vi "zlgcan_demo_PCIECANFD-200U.vi"() -> ()   [LabVIEW 2018]
doc: "用于设置CAN通道的初始化参数。\n\n适用的设备：PCIE-CANFD-100U、PCIE-CANFD-200U、PCIE-CANFD-400U。"
uses:
  data_type/ZCAN_Transmit_Data.ctl
  data_type/ZCAN_TransmitFD_Data.ctl
  data_type/ZCAN_InitCAN_setting_PCIEFD.ctl
panel:
  in  "PCIECANFD系列初始化参数":T1
  out "source":string
  in  "开启CAN":bool
  out "CANFD报文显示":string[][](table)
  in  "stop":bool
  in  "?":enum32{"DEMO说明", "设备、通道选择", "参数设置", "状态", "发送"}(tab)
  in  "CAN 通道":u32(ring) items=["0", "1"]
  in  "CAN卡型号":u32(ring)=39 items=["PCIE-CANFD-200U"=39]
  in  "索引":u32(ring) items=["0", "1", "2", "3", "4", "5", "6", "7", "8"]
  in  "仲裁域波特率":u32(ring)=500000 items=["1Mbps"=1000000, "800kbps"=800000, "500kbps"=500000, "250kbps"=250000, "125kbps"=125000, "100kbps"=100000, "50kbps"=50000]
  in  "数据域波特率":u32(ring)=1000000 items=["8Mbps"=8000000, "5Mbps"=5000000, "4Mbps"=4000000, "2Mbps"=2000000, "1Mbps"=1000000]
  in  "自定义波特率字符输入":string
  in  "自定义波特率开关":bool
  in  "验收码":u32
  in  "屏蔽码":u32=4294967295 format="%x"
  in  "滤波模式":u8(ring) items=["双滤波", "单滤波"]
  in  "工作模式":u8(ring) items=["正常", "只听"]
  out "error out":errorcluster caption="错误输出"
  out "can_index_handle(out)":u32
  out "Device_handle(out)":u32
  in  "帧类型":u32(ring) items=["标准帧", "扩展帧"]
  in  "发送方式":u32(ring) items=["正常发送", "单次发送", "自发自收", "单次自发自收"]
  in  "帧格式":u32(ring) items=["数据帧", "远程帧"]
  out "数据长度":u8=8 max=8
  in  "ID":u32=18 format="0x%08x"
  in  "协议":u32(ring) items=["CAN", "CANFD"]
  in  "数据输入":string="11 22 33 44 55 66 77 88"
  in  "CANFD加速？":u32(ring) items=["不加速", "加速"]
  in  "发送":bool
  in  "CANFD数据帧数组":T2(array[cluster])
  in  "CAN数据帧数组":T3(array[cluster])
  out "CAN报文显示":string[][](table)
  in  "ZCAN_TransmitFD_Data":T4
  in  "ZCAN_Transmit_Data":T5
  out "已接收帧数":u32
  # "适用的设备：PCIE-CANFD-200U。"
  # "停止程序前，\n请先关闭CAN卡"
  # "1. 确保电脑有VC++ 2005/2008/2010/2013运行库（对应32，64位）,微软常用运行库合集，点击下载（35M）。\n    http://manual.zlg.cn/Public/Uploads/2020-06-05/5ed995c271414.zip"
  # "2，如果打开设备失败，可能原因：\n（1）已经打开过一次，没有正常关闭的情况下，继续点击“打开设备”，是无法打开的。\n     需要USB重新拔插，LABVIEW重启（全部关闭），然后再“打开设备”。\n (2) 项目路径不能有中文繁体。"
  # "默认可以不设置"
  # "使用CAN时，\n只需要设置仲裁域波特率"
  # "使用ZCANPro软件波特率计算工具计算"
  # "CANFD数据长度只能是1~8，12，16，20，24，32，48，64"
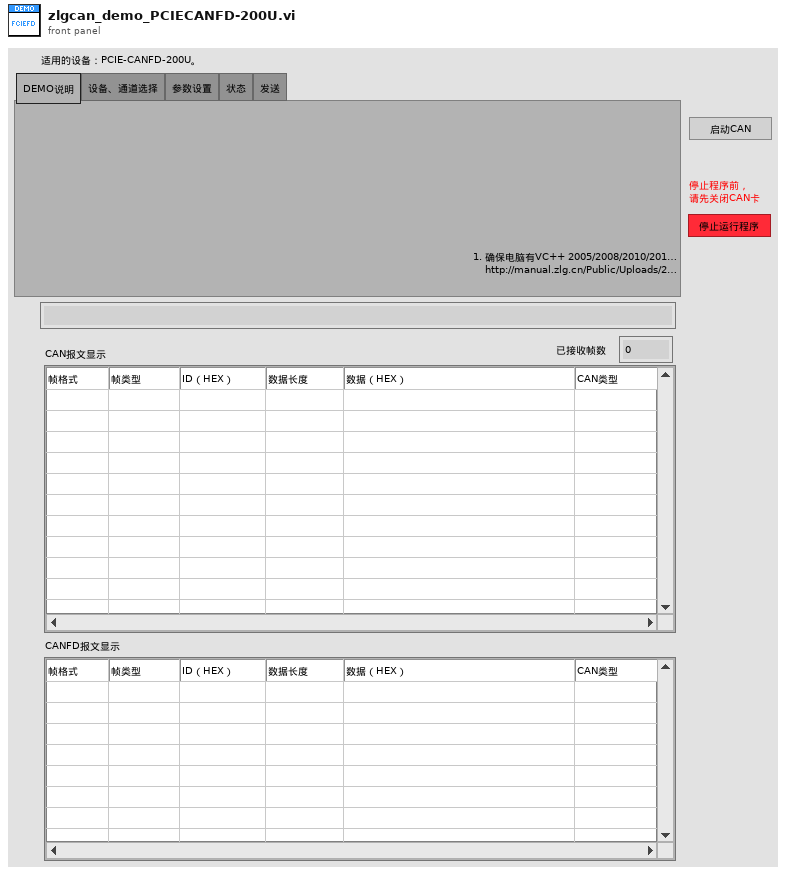
[diagram p1: front panel]
types:
  T1 = typedef "ZCAN_InitCAN_setting_PCIEFD.ctl" = cluster{"abitbaud":u32, "dbitbaud":u32, "baud_rate_custom？":bool, "RateCustom":string, "filter":u8, "acc_code":u32, "acc_mask":u32, "mode":u8}
  T2 = cluster{u32, u8, u8, u8, u8, cluster{"[0]":u8, "[1]":u8, "[2]":u8, "[3]":u8, "[4]":u8, "[5]":u8, "[6]":u8, "[7]":u8, "[8]":u8, "[9]":u8, "[10]":u8, "[11]":u8, "[12]":u8, "[13]":u8, "[14]":u8, "[15]":u8, "[16]":u8, "[17]":u8, "[18]":u8, "[19]":u8, "[20]":u8, "[21]":u8, "[22]":u8, "[23]":u8, "[24]":u8, "[25]":u8, "[26]":u8, "[27]":u8, "[28]":u8, "[29]":u8, "[30]":u8, "[31]":u8, "[32]":u8, "[33]":u8, "[34]":u8, "[35]":u8, "[36]":u8, "[37]":u8, "[38]":u8, "[39]":u8, "[40]":u8, "[41]":u8, "[42]":u8, "[43]":u8, "[44]":u8, "[45]":u8, "[46]":u8, "[47]":u8, "[48]":u8, "[49]":u8, "[50]":u8, "[51]":u8, "[52]":u8, "[53]":u8, "[54]":u8, "[55]":u8, "[56]":u8, "[57]":u8, "[58]":u8, "[59]":u8, "[60]":u8, "[61]":u8, "[62]":u8, "[63]":u8}, u64}[]
  T3 = cluster{u32, u8, u8, u8, u8, cluster{"[0]":u8, "[1]":u8, "[2]":u8, "[3]":u8, "[4]":u8, "[5]":u8, "[6]":u8, "[7]":u8}, u64}[]
  T4 = typedef "ZCAN_TransmitFD_Data.ctl" = cluster{"帧类型":u32, "帧格式":u32, "ID":u32, "数据长度":u8, "CANFD加速？":u8, "DATA":cluster{"CAN数据[0]":u8, "CAN数据[1]":u8, "CAN数据[2]":u8, "CAN数据[3]":u8, "CAN数据[4]":u8, "CAN数据[5]":u8, "CAN数据[6]":u8, "CAN数据[7]":u8, "CAN数据[8]":u8, "CAN数据[9]":u8, "CAN数据[10]":u8, "CAN数据[11] ":u8, "CAN数据[12] ":u8, "CAN数据[13] ":u8, "CAN数据[14] ":u8, "CAN数据[15] ":u8, "CAN数据[16]":u8, "CAN数据[17]":u8, "CAN数据[18]":u8, "CAN数据[19]":u8, "CAN数据[20]":u8, "CAN数据[21]":u8, "CAN数据[22]":u8, "CAN数据[23]":u8, "CAN数据[24] ":u8, "CAN数据[25]":u8, "CAN数据[26]":u8, "CAN数据[27]":u8, "CAN数据[28]":u8, "CAN数据[29]":u8, "CAN数据[30]":u8, "CAN数据[31]":u8, "CAN数据[32]":u8, "CAN数据[33]":u8, "CAN数据[34]":u8, "CAN数据[35]":u8, "CAN数据[36]":u8, "CAN数据[37]":u8, "CAN数据[38]":u8, "CAN数据[39]":u8, "CAN数据[40]":u8, "CAN数据[41]":u8, "CAN数据[42]":u8, "CAN数据[43]":u8, "CAN数据[44]":u8, "CAN数据[45]":u8, "CAN数据[46]":u8, "CAN数据[47]":u8, "CAN数据[48]":u8, "CAN数据[49]":u8, "CAN数据[50]":u8, "CAN数据[51]":u8, "CAN数据[52]":u8, "CAN数据[53]":u8, "CAN数据[54]":u8, "CAN数据[55]":u8, "CAN数据[56]":u8, "CAN数据[57]":u8, "CAN数据[58]":u8, "CAN数据[59]":u8, "CAN数据[60]":u8, "CAN数据[61]":u8, "CAN数据[62]":u8, "CAN数据[63]":u8}, "发送方式":u32}
  T5 = typedef "ZCAN_Transmit_Data.ctl" = cluster{"帧类型":u32, "帧格式":u32, "ID":u32, "数据长度":u8, "DATA":cluster{"CAN数据[0]":u8, "CAN数据[1]":u8, "CAN数据[2]":u8, "CAN数据[3]":u8, "CAN数据[4]":u8, "CAN数据[5]":u8, "CAN数据[6]":u8, "CAN数据[7]":u8}, "发送方式":u32}
  T6 = cluster{"[0]":u32, "[1]":u32, "[2]":u32, "[3]":u32, "[4]":u32, "[5]":u32, "[6]":u32, "[7]":u32, "[8]":u32, "[9]":u32, "[10]":u32, "[11]":u32, "[12]":u32, "[13]":u32, "[14]":u32, "[15]":u32, "[16]":u32, "[17]":u32, "[18]":u32, "[19]":u32, "[20]":u32, "[21]":u32, "[22]":u32, "[23]":u32, "[24]":u32, "[25]":u32, "[26]":u32, "[27]":u32, "[28]":u32, "[29]":u32, "[30]":u32, "[31]":u32, "[32]":u32, "[33]":u32, "[34]":u32, "[35]":u32, "[36]":u32, "[37]":u32, "[38]":u32, "[39]":u32, "[40]":u32, "[41]":u32, "[42]":u32, "[43]":u32, "[44]":u32, "[45]":u32, "[46]":u32, "[47]":u32, "[48]":u32, "[49]":u32, "[50]":u32, "[51]":u32, "[52]":u32, "[53]":u32, "[54]":u32, "[55]":u32, "[56]":u32, "[57]":u32, "[58]":u32, "[59]":u32, "[60]":u32, "[61]":u32, "[62]":u32, "[63]":u32}
  T7 = cluster{"[0]":u32, "[1]":u32, "[2]":u32, "[3]":u32, "[4]":u32, "[5]":u32, "[6]":u32, "[7]":u32}
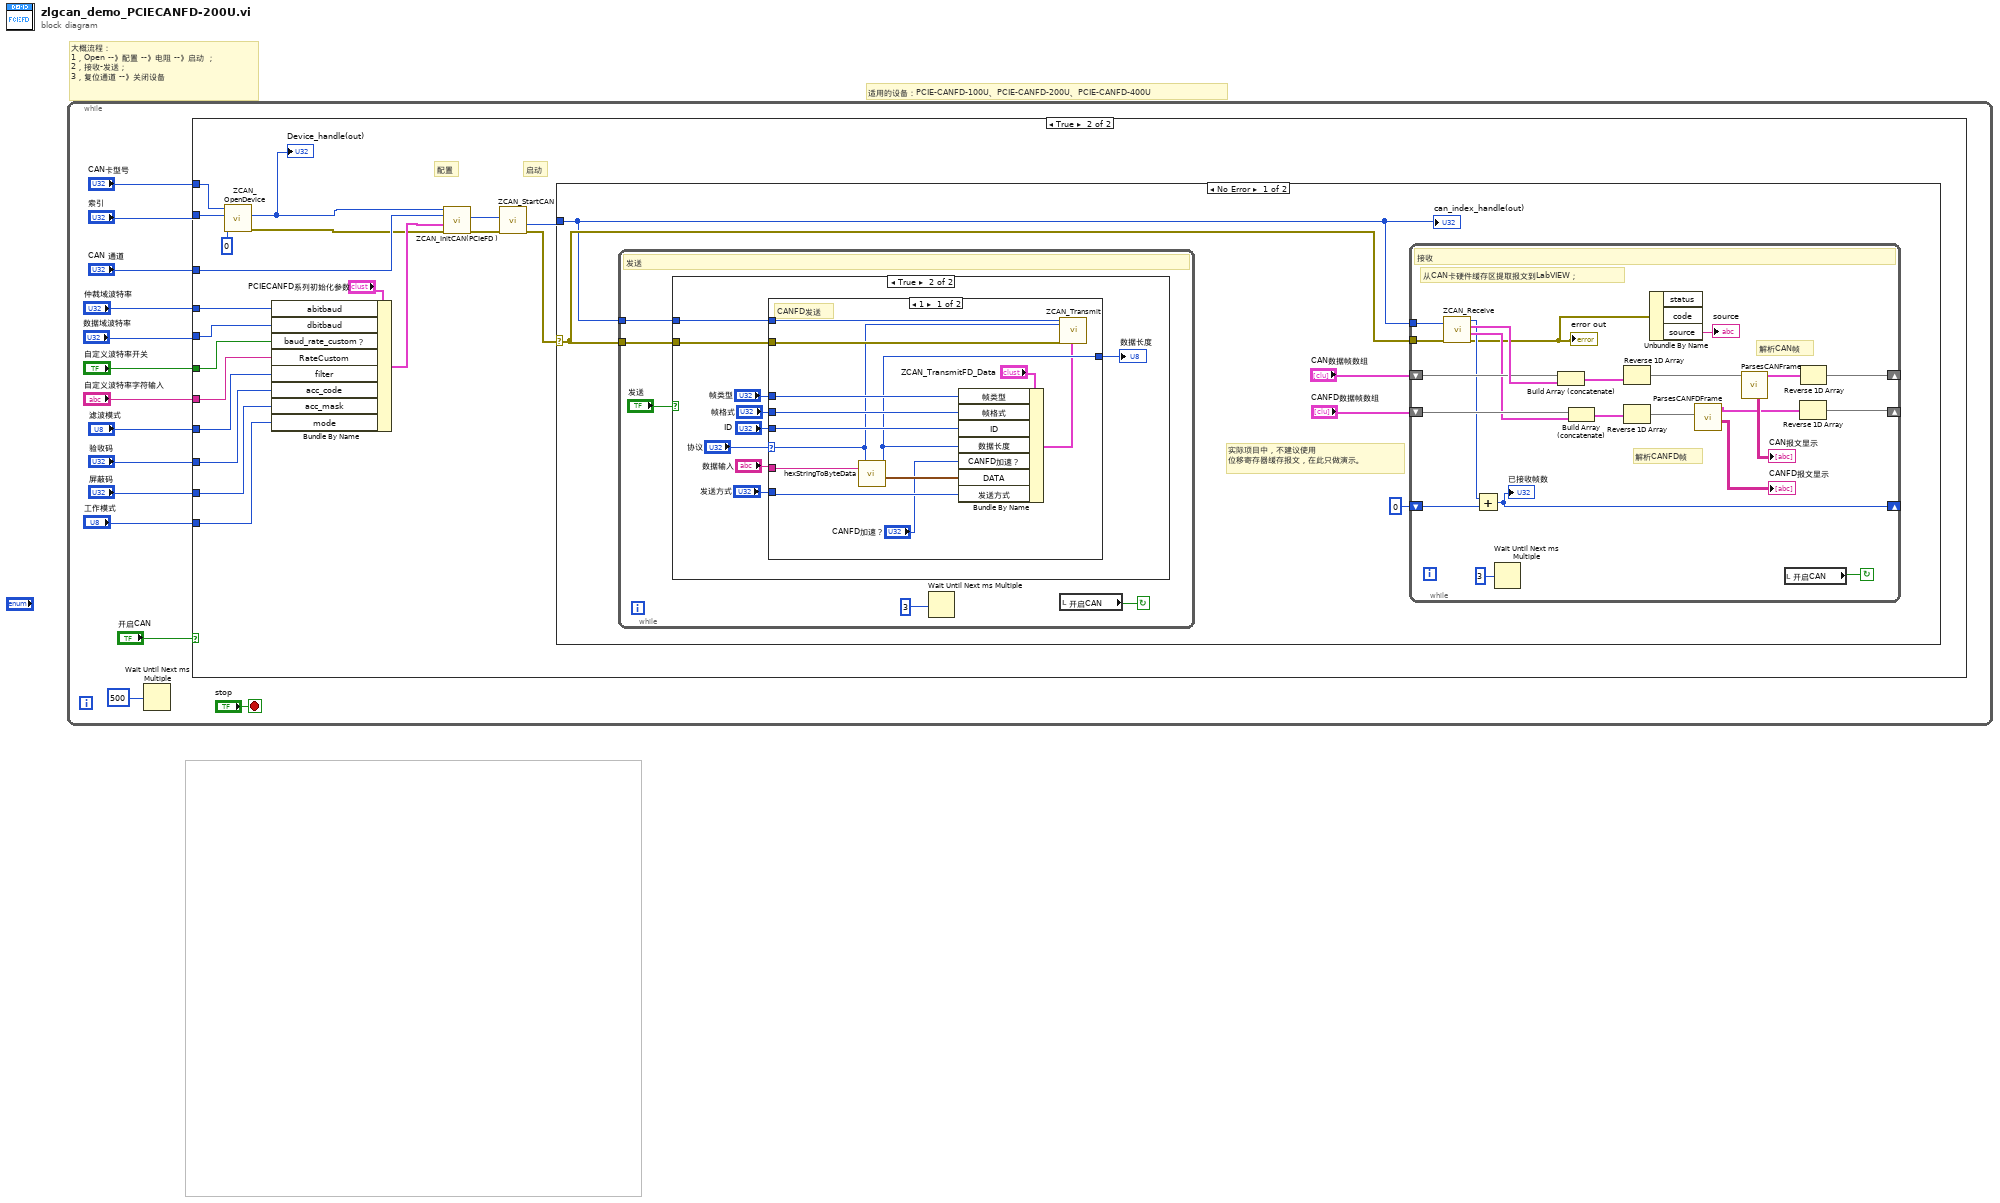
[diagram p0: block diagram]
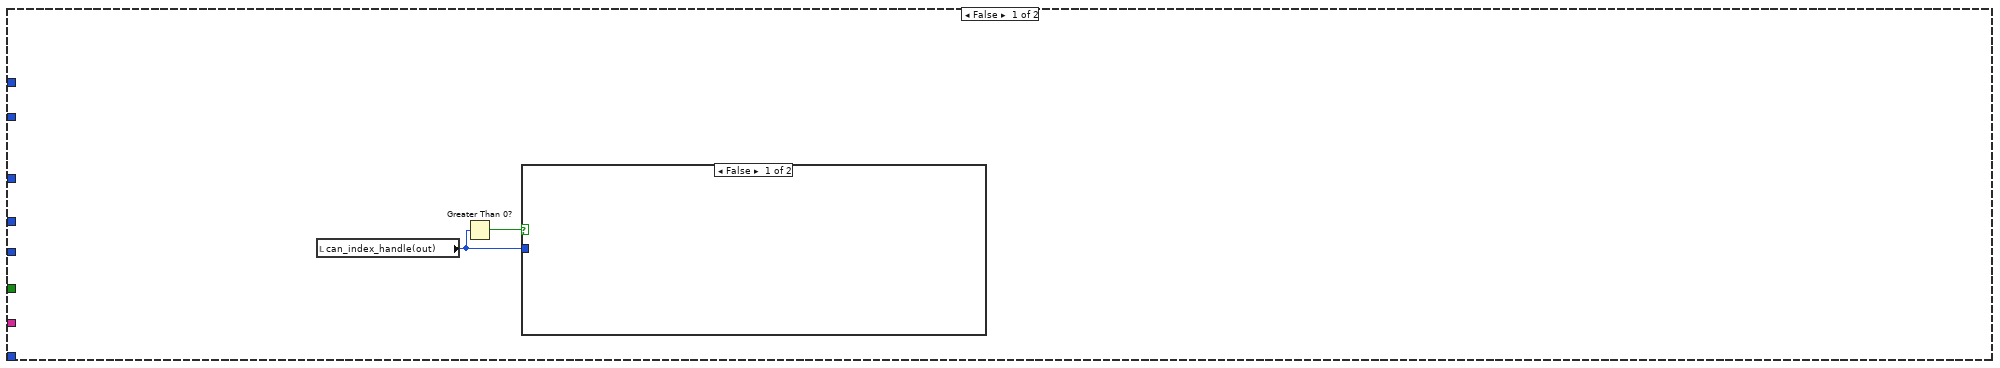
[diagram p2: hidden frame]
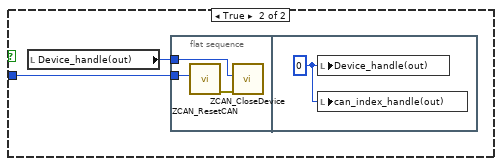
[diagram p3: hidden frame]
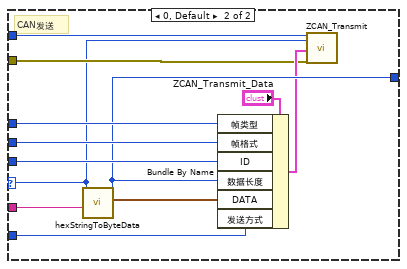
[diagram p5: hidden frame]
diagram:
  # "大概流程：\n1，Open --》配置 --》电阻 --》启动 ；\n2，接收-发送；\n3，复位通道 --》关闭设备"
  # "适用的设备：PCIE-CANFD-100U、PCIE-CANFD-200U、PCIE-CANFD-400U"
  n1 = while {
    stop <- "stop" stop-if-true
    n2 = Wait Until Next ms Multiple(millisecond multiple=u32 500) -> ()  [unwired: 1 out]
    n3 = case shown="True" "开启CAN" {
      tunnel: "CAN 通道" -> [_ w31]
      tunnel: "仲裁域波特率" -> [_ w36]
      tunnel: "自定义波特率开关" -> [_ w38]
      tunnel: "自定义波特率字符输入" -> [_ w35]
      tunnel: "工作模式" -> [_ w25]
      tunnel: "CAN卡型号" -> [_ w40]
      tunnel: "索引" -> [_ w41]
      tunnel: "数据域波特率" -> [_ w37]
      tunnel: "滤波模式" -> [_ w28]
      tunnel: "验收码" -> [_ w27]
      tunnel: "屏蔽码" -> [_ w26]
      frame False {
        # "关闭CAN卡"
        n4 = local read "can_index_handle(out)"() -> (w15:u32)
        n5 = Greater Than 0?(x=w15) -> (x > 0?=w16:bool)
        n6 = case shown="False" w16 {
          tunnel: w15 -> [_ w18]
          frame False {
          }
          frame True {
            n7 = local read "Device_handle(out)"() -> (w17:u32)
            n8 = flat-sequence {
              tunnel: w18 -> [w20]
              tunnel: w17 -> [w19]
              frame #0 {
                n9 = call "ZCAN_ResetCAN.vi"("can_handle"=w20) -> ("error out"=w21:errorcluster)  [unwired: 9 in, 1 out]
                n10 = call "ZCAN_CloseDevice.vi"("error in (no error)"=w21, "device_handle"=w19) -> ()  [unwired: 8 in, 2 out]
              }
              frame #1 {
                w22 = u32 0 ("can_index_handle(out)")
                n11 = local write "Device_handle(out)"(w22) -> ()
                n12 = local write "can_index_handle(out)"(w22) -> ()
              }
            }
          }
        }
      }
      frame True {
        # "启动"
        # "配置"
        n13 = call "ZCAN_OpenDevice.vi"("reserved"=0, "device_index"=w41, "device_type"=w40) -> ("error out"=w23:errorcluster, "DEVICE_HANDLE"=w24:u32)  [unwired: 7 in]
        "Device_handle(out)" <- w24
        n14 = Bundle By Name(cluster="PCIECANFD系列初始化参数", "abitbaud"=w36, "dbitbaud"=w37, "baud_rate_custom？"=w38, "RateCustom"=w35, "filter"=w28, "acc_code"=w27, "acc_mask"=w26, "mode"=w25) -> (w30:T1)
        n15 = call "ZCAN_InitCAN(PCIeFD ).vi"("error in (no error)"=w23, "PCIECANFD系列初始化参数"=w30, "can_index"=w31, "device_hande"=w24) -> ("error out"=w33:errorcluster, "can_index_handle"=w32:u32)  [unwired: 2 in]
        n16 = call "ZCAN_StartCAN.vi"("error in (no error)"=w33, "can_index_handle"=w32) -> ("error out"=w34:errorcluster, "can_index_handle(out)"=w39:u32)  [unwired: 7 in, 1 out]
        n17 = case shown="No Error" w34 {
          selector: w34 -> [w46 _]
          tunnel: w39 -> [w45 _]
          frame No Error {
            # "实际项目中，不建议使用\n位移寄存器缓存报文，在此只做演示。"
            n18 = while {
              tunnel: w45 -> [w73]
              tunnel: w46 -> [w71]
              stop <- w72 continue-if-true
              # "发送"
              n19 = case shown="True" "发送" {
                tunnel: w73 -> [_ w77]
                tunnel: w71 -> [_ w78]
                frame False {
                }
                frame True {
                  n20 = case shown="1" "协议" {
                    selector: "协议" -> [w85 w98]
                    tunnel: "帧类型" -> [w96 w108]
                    tunnel: "帧格式" -> [w95 w107]
                    tunnel: "ID" -> [w94 w106]
                    tunnel: "发送方式" -> [w93 w104]
                    tunnel: [w89 w103] -> w79
                    tunnel: "数据输入" -> [w91 w102]
                    tunnel: w78 -> [w88 w100]
                    tunnel: w77 -> [w86 w99]
                    frame 1 {
                      # "CANFD发送"
                      n21 = call "hexStringToByteData.vi"("数据输入"=w91, "协议"=w85) -> ("CANFD_data"=w92:T6, "字节数"=w89:i32)  [unwired: 7 in, 1 out]
                      n22 = Bundle By Name(cluster="ZCAN_TransmitFD_Data", "帧类型"=w96, "帧格式"=w95, "ID"=w94, "数据长度"=w89, "CANFD加速？"="CANFD加速？", "DATA"=w92, "发送方式"=w93) -> (w87:T4)
                      n23 = call "ZCAN_Transmit.vi"("can_index_handle"=w86, "协议"=w85, "error in (no error)"=w88, "ZCAN_TransmitFD_Data"=w87) -> ()  [unwired: 15 in, 1 out]
                    }
                    frame 0, Default {
                      # "CAN发送"
                      n24 = call "hexStringToByteData.vi"("数据输入"=w102, "协议"=w98) -> ("CAN_data"=w105:T7, "字节数"=w103:i32)  [unwired: 7 in, 1 out]
                      n25 = Bundle By Name(cluster="ZCAN_Transmit_Data", "帧类型"=w108, "帧格式"=w107, "ID"=w106, "数据长度"=w103, "DATA"=w105, "发送方式"=w104) -> (w101:T5)
                      n26 = call "ZCAN_Transmit.vi"("can_index_handle"=w99, "协议"=w98, "ZCAN_Transmit_Data"=w101, "error in (no error)"=w100) -> ()  [unwired: 15 in, 1 out]
                    }
                  }
                  "数据长度" <- w79
                }
              }
              n27 = Wait Until Next ms Multiple(millisecond multiple=u32 3) -> ()  [unwired: 1 out]
              n28 = local read "开启CAN"() -> (w72:bool)
            }
            n29 = while {
              tunnel: w46 -> [w68]
              tunnel: w45 -> [w67]
              shift-right: [w69] -> _
              shift-left: 0 -> [w54]
              shift-right: [w58] -> _
              shift-left: "CAN数据帧数组" -> [w64]
              shift-right: [w56] -> _
              shift-left: "CANFD数据帧数组" -> [w62]
              stop <- w66 continue-if-true
              # "从CAN卡硬件缓存区提取报文到LabVIEW；"
              # "解析CANFD帧"
              # "解析CAN帧"
              # "接收"
              n30 = call "ZCAN_Receive.vi"("error in (no error)"=w68, "can_handle"=w67) -> ("error out"=w48:errorcluster, "CANFD数据帧数组"=w61:T2, "CAN数据帧数组"=w65:T3, "Receive_Num"=w55:u32)  [unwired: 2 in]
              "error out" <- w48
              n31 = Add(x=w55, y=w54) -> (x+y=w69:u32)
              "已接收帧数" <- w69
              n32 = Wait Until Next ms Multiple(millisecond multiple=u32 3) -> ()  [unwired: 1 out]
              n33 = Build Array (concatenate)(w64, w65) -> (w63:T3)
              n34 = Build Array (concatenate)(w62, w61) -> (w60:T2)
              n35 = Reverse 1D Array(array=w63) -> (reversed array=w57:T3)
              n36 = Reverse 1D Array(array=w60) -> (reversed array=w52:T2)
              n37 = Unbundle By Name(w48) -> ("source"=→"source":string)  [unwired: 2 out]
              n38 = call "ParsesCANFDFrame.vi"("CANFD数据帧数组"=w52) -> ("CANFD报文显示"=→"CANFD报文显示":string[][], "CANFD数据帧数组(out)"=w51:T2)  [unwired: 9 in]
              n39 = call "ParsesCANFrame.vi"("CAN数据帧数组"=w57) -> ("CAN数据帧数组(out)"=w59:T3, "CAN报文显示"=→"CAN报文显示":string[][])  [unwired: 9 in]
              n40 = local read "开启CAN"() -> (w66:bool)
              n41 = Reverse 1D Array(array=w51) -> (reversed array=w56:T2)
              n42 = Reverse 1D Array(array=w59) -> (reversed array=w58:T3)
            }
            "can_index_handle(out)" <- w45
          }
          frame Error {
          }
        }
      }
    }
  }
